vi "OneTouchShotTest.vi"(0 "object in":refnum<class "Game.lvclass">, 2 "grSimReplacement":T1, 4 "start":bool=TRUE, 5 "error in (no error)":errorcluster) -> (14 "object out":refnum<class "Game.lvclass">, 16 "TestTeam out":refnum<class "Ally.lvclass">, 18 "grSImReplacement out":T1, 19 "error out":errorcluster)   [LabVIEW 2023, in "Game.lvclass"]
uses:
  Game.lvclass
  Communication_class/Paths/grSim Packet Command UDP Test Folder/grSim/grSim_BallReplacement.ctl
  Ally_class/Ally.lvclass
  Controls/grSimReplacement.ctl
  Communication_class/Paths/grSim Packet Command UDP Test Folder/grSim/grSim RobotReplacement.ctl
  Game.lvclass/Game.ctl
  Team_class/Team.lvclass/Team.ctl
  Robot_class/Robot.lvclass/Robot.ctl
  Object_class/Object.lvclass/Object.ctl
  <vilib>/Analysis/baseanly.llb/Unit Vector (DBL).vi
  Object_class/Read position(x,y).vi
  Team_class/Read RobotRef.vi
  Robot_class/Write kick_x.vi
  Team_class/Write RobotRef.vi
  Read TestTeam.vi
  Read AllyRef.vi
  Read BallRef.vi
  Ball_class/Ball.lvclass
  Robot_class/Robot.lvclass
  <vilib>/Analysis/NI_AALBase.lvlib
panel:
  in  "xline":dbl=176.327 format="%#_13g"
  in  "ball":T3
  out "Desvio":dbl[](array[numeric])
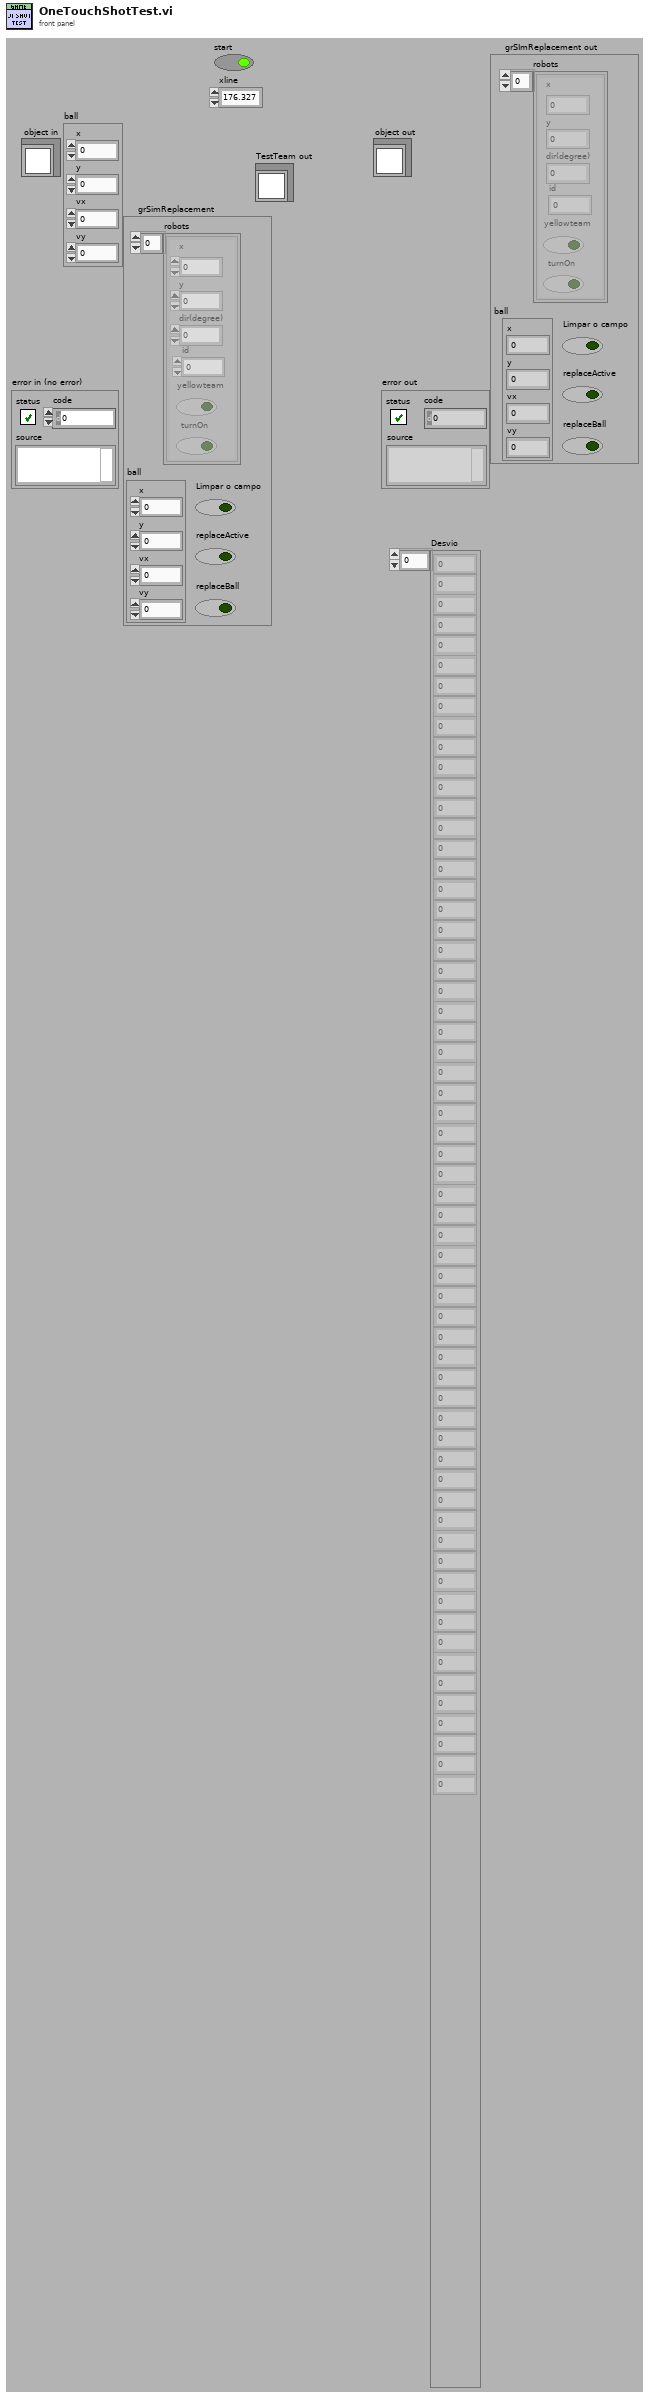
[diagram p1: front panel]
types:
  T1 = typedef "grSimReplacement.ctl" = cluster{"robots":T2[], "ball":T3, "replaceBall":bool, "replaceActive":bool, "Limpar o campo":bool}
  T2 = typedef "grSim RobotReplacement.ctl" = cluster{"x":dbl, "y":dbl, "dir(degree)":dbl, "yellowteam":bool, "id":u32, "turnOn":bool}
  T3 = typedef "grSim_BallReplacement.ctl" = cluster{"x":dbl, "y":dbl, "vx":dbl, "vy":dbl}
  T4 = typedef "STPParameters.ctl" = cluster{"Skills":T5, "TestSkill":T7, "Events":cluster{"distanceToBallPossession":dbl, "timeForPossessionThreshold":dbl}, "Criteria":cluster{"OpenAngleToGoal":cluster{"minAngle":dbl, "maxAngle":dbl, "minEvaluation":dbl}, "PassDistance":cluster{"maxDistance":dbl, "minDistance":dbl}, "ShotInterception":cluster{"shotSpeed":dbl, "minEnemySpeed":dbl, "minEvaluation":dbl, "maxEnemySpeed":dbl}, "OneTouchShot":cluster{"MaxAngle":dbl, "minEvaluation":dbl}, "PassInterception":cluster{"minEnemySpeed":dbl, "maxEnemySpeed":dbl, "chipPassDistance":dbl, "chipPassEval":dbl, "minEvaluation":dbl}}, "minPassSpeed":dbl, "maxPassSpeed":dbl, "AllyTeamIds":T8[], "ReceiverSpeed":dbl, "minEvaluationToShoot":dbl, "maxDefendersNumber":u8, "slackTime":dbl}
  T5 = typedef "Skills.ctl" = cluster{"CirculateBall":T6, "ProtectBall":cluster{"DistanceFromBall":dbl}}
  T6 = typedef "CIrculateSkillParameters.ctl" = cluster{"rotationAngle":dbl, "velocityFactor":dbl, "OrientationFactor":dbl}
  T7 = typedef "TestSkills.ctl" = enum16{"AlignSkill", "PassSkill", "CirculateBall", "OneTouchShotSkill", "KickToSkill_v2", "ShootSkill", "InterceptBall", "Exit", "GoToSkill_v2"}
  T8 = typedef "AllyTeam.ctl" = enum16{"Keeper", "Defender", "Attacker"}
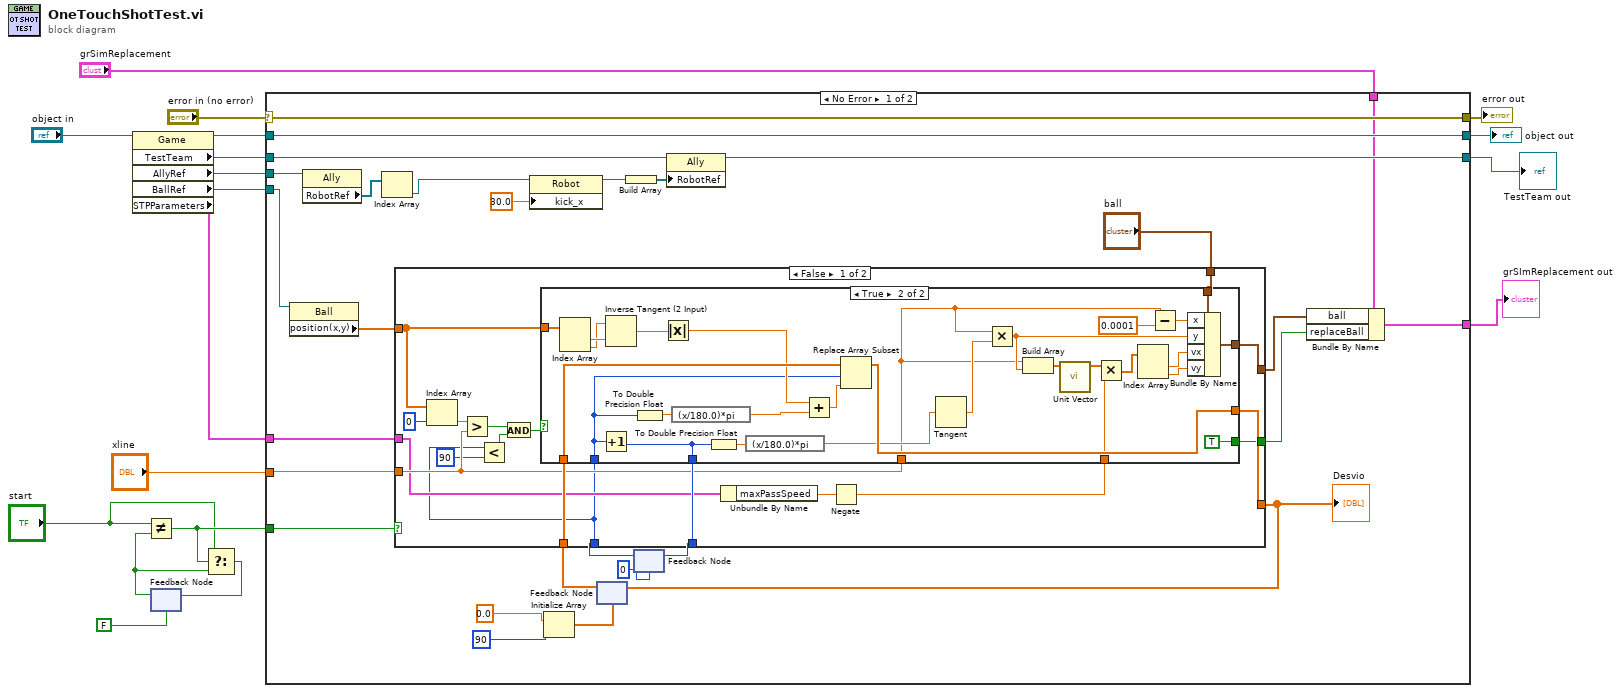
[diagram p0: block diagram]
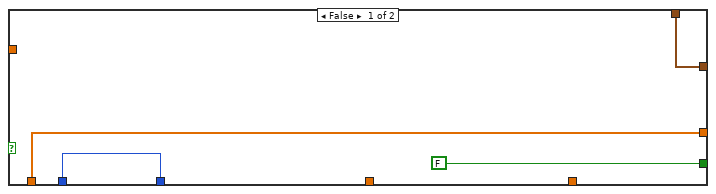
[diagram p2: hidden frame]
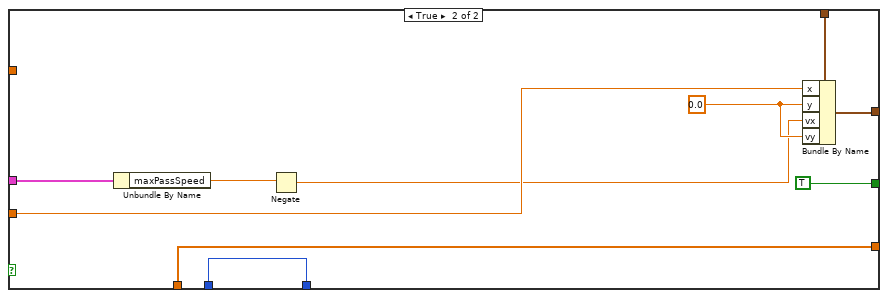
[diagram p3: hidden frame]
diagram:
  n1 = property class="Game"(reference="object in") -> (reference out=w9:refnum<class "Game.lvclass">, "TestTeam"=w13:refnum<class "Ally.lvclass">, "AllyRef"=w12:refnum<class "Ally.lvclass">, "BallRef"=w11:refnum<class "Ball.lvclass">, "STPParameters"=w6:T4)  [unwired: 1 in, 1 out]
  n2 = feedback #1(FALSE ("start")) -> (w2:bool)
  n3 = Not Equal?(x="start", y=w2) -> (x != y?=w4:bool)
  n4 = Select(t="start", s=w4, f=w2) -> (s? t:f=w3:bool)
  n5 = feedback-in #1(w3) -> ()
  n6 = case shown="No Error" "error in (no error)" {
    selector: "error in (no error)" -> [w46 w110]
    tunnel: [w46 w110] -> w17
    tunnel: [w31 w109] -> w15
    tunnel: w9 -> [w31 w109]
    tunnel: [w30 w107] -> w14
    tunnel: w13 -> [w29 w107]
    tunnel: w12 -> [w28 _]
    tunnel: w11 -> [w27 _]
    tunnel: [w26 w108] -> w10
    tunnel: "grSimReplacement" -> [w25 w108]
    tunnel: "xline" -> [w24 _]
    tunnel: w6 -> [w23 _]
    tunnel: w4 -> [w22 _]
    frame No Error {
      n7 = property class="Ball"(reference=w27) -> ("position(x,y)"=w40:dbl[])  [unwired: 1 in, 2 out]
      n8 = property class="Ally"(reference=w28) -> ("RobotRef"=w45:refnum<class "Robot.lvclass">[])  [unwired: 1 in, 2 out]
      n9 = Index Array(array=w45) -> (element=w44:refnum<class "Robot.lvclass">)  [unwired: 1 in]
      n10 = property class="Robot"(reference=w44, "kick_x"=30.0) -> (reference out=w42:refnum<class "Robot.lvclass">)  [unwired: 1 in, 1 out]
      n11 = Initialize Array(0.0 ("element"), 90 ("dimension size")) -> (w39:dbl[])
      n12 = feedback #2(w39) -> (w37:dbl[])
      n13 = Build Array(w42) -> (w41:refnum<class "Robot.lvclass">[])
      n14 = feedback #3(0) -> (w20:i32)
      n15 = case shown="False" w22 {
        tunnel: w40 -> [w63 _]
        tunnel: w37 -> [w61 w102]
        tunnel: [w60 w102] -> w36
        tunnel: [w59 TRUE] -> w35
        tunnel: [w58 w104] -> w33
        tunnel: "ball" -> [w57 w105]
        tunnel: w24 -> [w55 w100]
        tunnel: w23 -> [w54 w103]
        tunnel: w20 -> [w49 w101]
        tunnel: [w56 w101] -> w19
        frame False {
          n16 = Index Array(array=w63, index=0) -> (element=w64:dbl)
          n17 = Greater?(x=w64, y=w55) -> (0:w51:bool)
          n18 = Less?(x=w49, y=90) -> (x < y?=w47:bool)
          n19 = And(x=w51, y=w47) -> (x .and. y?=w50:bool)
          n20 = Unbundle By Name(w54) -> ("maxPassSpeed"=w53:dbl)
          n21 = Negate(x=w53) -> (-x=w52:dbl)
          n22 = case shown="True" w50 {
            tunnel: w63 -> [_ w96]
            tunnel: w49 -> [w68 w84]
            tunnel: w61 -> [w67 w93]
            tunnel: [w67 w91] -> w60
            tunnel: [w68 w81] -> w56
            tunnel: [FALSE TRUE] -> w59
            tunnel: [w65 w90] -> w58
            tunnel: w57 -> [w65 w89]
            tunnel: w55 -> [_ w71]
            tunnel: w52 -> [_ w78]
            frame False {
            }
            frame True {
              n23 = Index Array(array=w96) -> (element #1=w95:dbl, element #2=w94:dbl)  [unwired: 2 in]
              n24 = Increment(x=w84) -> (x+1=w81:i32)
              n25 = Inverse Tangent (2 Input)(1:w95, 2:w94) -> (0:w87:dbl)
              n26 = To Double Precision Float(number=w84) -> (double precision float=w85:dbl)
              n27 = Absolute Value(x=w87) -> (abs(x)=w86:dbl)
              n28 = expression code="(x/180.0)*pi" ("degrees to radians")(w85) -> (w83:dbl)
              n29 = To Double Precision Float(number=w81) -> (double precision float=w82:dbl)
              n30 = expression code="(x/180.0)*pi" ("degrees to radians")(w82) -> (w80:dbl)
              n31 = Add(x=w86, y=w83) -> (x+y=w88:dbl)
              n32 = Replace Array Subset(array=w93, new element=w88, index=w84) -> (w91:dbl[])
              n33 = Tangent(1:w80) -> (0:w79:dbl)
              n34 = Multiply(x=w71, y=w79) -> (x*y=w72:dbl)
              n35 = Build Array(w71, w72) -> (w75:dbl[])
              n36 = call-poly <vilib>:"Unit Vector.vi"("Input Vector"=w75) -> ("Unit Vector"=w73:dbl[])  [unwired: 8 in, 2 out]
              n37 = Multiply(x=w73, y=w78) -> (x*y=w74:dbl[])
              n38 = Index Array(array=w74) -> (element #1=w76:dbl, element #2=w77:dbl)  [unwired: 2 in]
              n39 = Subtract(x=w71, y=0.0001) -> (x-y=w69:dbl)
              n40 = Bundle By Name(cluster=w89, "x"=w69, "y"=w72, "vx"=w76, "vy"=w77) -> (w90:T3)
            }
          }
        }
        frame True {
          w99 = 0.0 ("y")
          n41 = Unbundle By Name(w103) -> ("maxPassSpeed"=w98:dbl)
          n42 = Negate(x=w98) -> (-x=w97:dbl)
          n43 = Bundle By Name(cluster=w105, "x"=w100, "y"=w99, "vx"=w97, "vy"=w99) -> (w104:T3)
        }
      }
      "Desvio" <- w36
      n44 = feedback-in #2(w36) -> ()
      n45 = feedback-in #3(w19) -> ()
      n46 = property class="Ally"(reference=w29, "RobotRef"=w41) -> (reference out=w30:refnum<class "Ally.lvclass">)  [unwired: 1 in, 1 out]
      n47 = Bundle By Name(cluster=w25, "ball"=w33, "replaceBall"=w35) -> (w26:T1)
    }
    frame Error {
    }
  }
  "error out" <- w17
  "object out" <- w15
  "TestTeam out" <- w14
  "grSImReplacement out" <- w10
